vi "Write Rooms.vi"(8 "error in (no error)":errorcluster, 10 "Rooms":T1, 11 "Door":refnum<class "Door.lvclass">) -> (0 "error out":errorcluster, 3 "Door":refnum<class "Door.lvclass">)   [LabVIEW 2020, in "Door.lvclass"]
uses:
  Door.lvclass
  Room/Room.lvclass
  Door.lvclass/Door.ctl
  TypeDef/privateDataDVR.ctl
  TypeDef/privateData.ctl
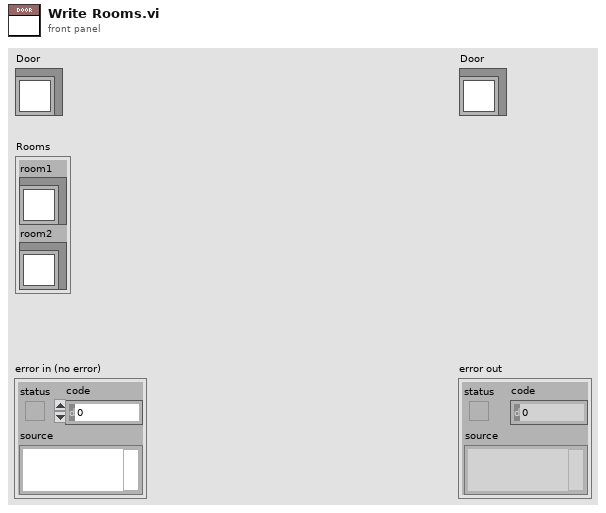
[diagram p1: front panel]
types:
  T1 = cluster{"room1":refnum<class "Room.lvclass">, "room2":refnum<class "Room.lvclass">}
  T2 = typedef "Door.lvclass/privateDataDVR.ctl" = refnum<data-value>
  T3 = typedef "Door.lvclass/privateData.ctl" = cluster{"room1":refnum<class "Room.lvclass">, "room2":refnum<class "Room.lvclass">}
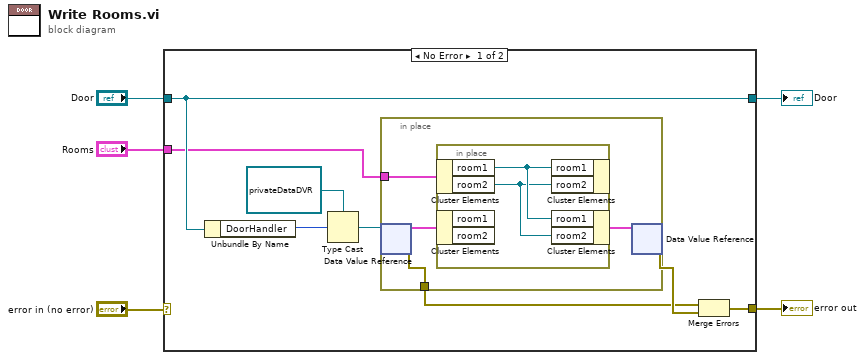
[diagram p0: block diagram]
diagram:
  n1 = case shown="No Error" "error in (no error)" {
    selector: "error in (no error)" -> [_ w20]
    tunnel: "Door" -> [w9 w21]
    tunnel: [w9 w21] -> w4
    tunnel: [w8 w20] -> w3
    tunnel: "Rooms" -> [w6 _]
    frame No Error {
      n2 = Unbundle By Name(w9) -> ("DoorHandler"=w11:u32)
      n3 = Type Cast(type=T2 refnum ("privateDataDVR"), x=w11) -> (*(type *) &x=w13:T2)
      n4 = in-place {
        in-place-border: [w16] -> w10
        in-place-border: w6 -> [w14]
        n5 = in-place-dvr #1(w13) -> (w17:T3, w16:errorcluster)
        n6 = in-place {
          n7 = in-place-cluster #2(w14) -> ("room1"=w19:refnum<class "Room.lvclass">, "room2"=w18:refnum<class "Room.lvclass">)
          n8 = in-place-cluster #3(w17) -> ()  [unwired: 2 out]
          n9 = in-place-cluster #2("room1"=w19, "room2"=w18) -> ()  [unwired: 1 out]
          n10 = in-place-cluster #3("room1"=w19, "room2"=w18) -> (w15:T3)
        }
        n11 = in-place-dvr #1(w15) -> (w12:errorcluster)  [unwired: 1 out]
      }
      n12 = Merge Errors(w10, w12) -> (w8:errorcluster)
    }
    frame Error {
    }
  }
  "error out" <- w3
  "Door" <- w4
